vi "Off.vi"(8 "error in (no error)":errorcluster, 11 "LED in":refnum<class "LED.lvclass">) -> (0 "error out":errorcluster, 3 "LED out":refnum<class "LED.lvclass">)   [LabVIEW 2016, in "LED.lvclass"]
uses:
  LED.lvclass
  LightBox/LightBox.lvclass
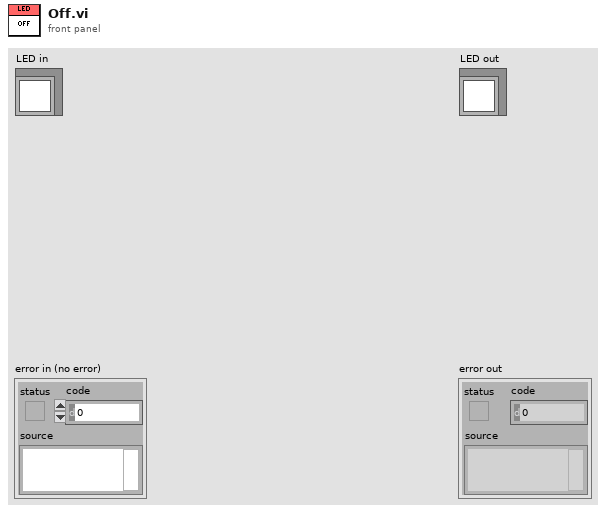
[diagram p1: front panel]
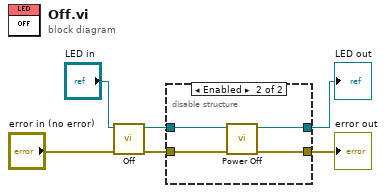
[diagram p0: block diagram]
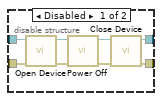
[diagram p2: hidden frame]
diagram:
  n1 = call-parent "Off.vi"("error in (no error)"="error in (no error)", "Lamp in"="LED in") -> ("error out"=w1:errorcluster, "Lamp out"=w2:refnum<class "LED.lvclass">)  [unwired: 8 in]
  n2 = disable-structure shown="Enabled" {
    disable-tunnel: [w12 w16] -> w4
    disable-tunnel: [w11 w17] -> w3
    disable-tunnel: w2 -> [w8 w18]
    disable-tunnel: w1 -> [w7 w15]
    frame Disabled {
      n3 = call-dynamic "Open Device.vi"("error in (no error)"=w7, "LightBox in"=w8) -> ("error out"=w9:errorcluster, "LightBox out"=w10:refnum<class "LED.lvclass">)  [unwired: 8 in]
      n4 = call "Power Off.vi"("error in (no error)"=w9, "LED in"=w10) -> ("error out"=w13:errorcluster, "LED out"=w14:refnum<class "LED.lvclass">)  [unwired: 8 in]
      n5 = call-dynamic "Close Device.vi"("error in (no error)"=w13, "LightBox in"=w14) -> ("error out"=w12:errorcluster, "LightBox out"=w11:refnum<class "LED.lvclass">)  [unwired: 8 in]
    }
    frame Enabled {
      n6 = call "Power Off.vi"("error in (no error)"=w15, "LED in"=w18) -> ("error out"=w16:errorcluster, "LED out"=w17:refnum<class "LED.lvclass">)  [unwired: 8 in]
    }
  }
  "error out" <- w4
  "LED out" <- w3
